vi "Get Cal Proc List.vi"(6 "교정절차 목록 MC List":refnum<vi>, 8 "에러 입력(에러 없음)":errorcluster, 10 "교정정보 in":T1, 11 "참조 번호 입력":T2) -> (0 "에러 출력":errorcluster, 3 "참조 번호 출력":T2, 5 "교정정보 out":T1)   [LabVIEW 2020]
uses:
  <vilib>/addons/database/Connection.llb/Conn ObjectReference.ctl
  Controls/Clst_Cal Info Global.ctl
  Controls/Cmd_Read Query.ctl
  Controls/Clst_Query Info.ctl
  <vilib>/addons/database/NI_Database_API.lvlib
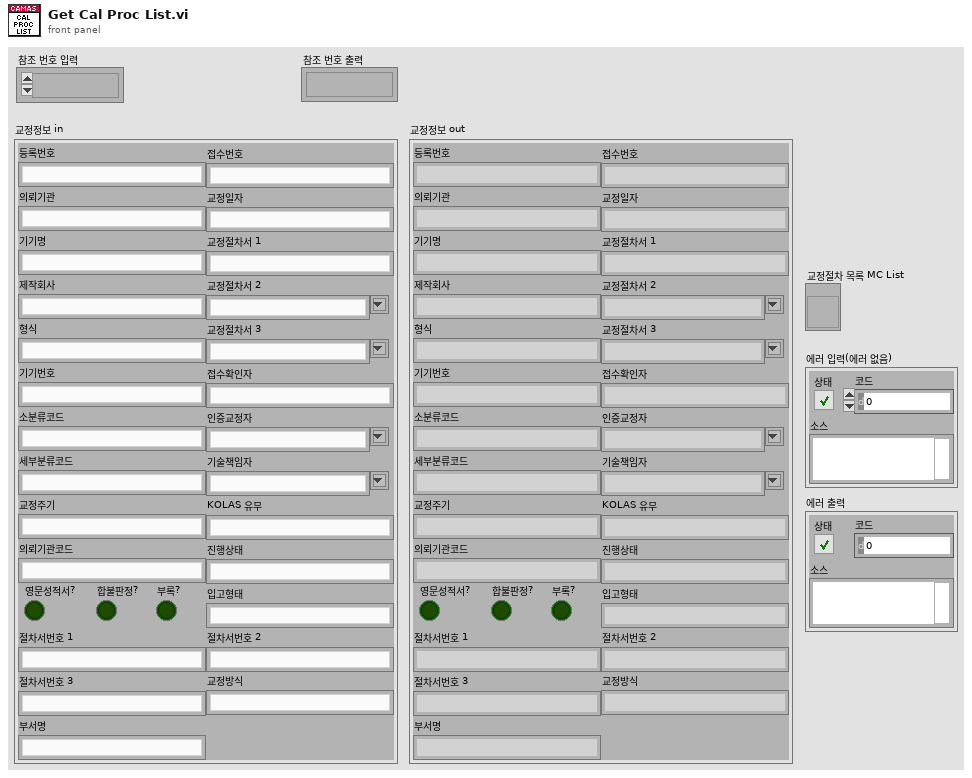
[diagram p1: front panel]
types:
  T1 = typedef "Clst_Cal Info Global.ctl" = cluster{"등록번호":string, "의뢰기관":string, "기기명":string, "제작회사":string, "형식":string, "기기번호":string, "소분류코드":string, "세부분류코드":string, "교정주기":string, "접수번호":string, "교정일자":string, "교정절차서 1":string, "교정절차서 2":string, "교정절차서 3":string, "접수확인자":string, "인증교정자":string, "기술책임자":string, "KOLAS 유무":string, "진행상태":string, "의뢰기관코드":string, "입고형태":string, "영문성적서?":bool, "합불판정?":bool, "부록?":bool, "절차서번호 1":string, "절차서번호 2":string, "절차서번호 3":string, "교정방식":string, "부서명":string}
  T2 = typedef "NI_Database_API.lvlib/Conn ObjectReference.ctl" = refnum<k1>
  T3 = typedef "Clst_Query Info.ctl" = cluster{"사번":string, "등록번호":string, "업체명":string, "세부분류코드":string, "형식":string, "기기번호":string, "FUNC":string, "FUNC_EXT":string, "옵션":string, "추가문자열":string, "일자":string, "배열 1":string[], "배열 2":string[], "항목명":string, "문자열":string, "이름":string}
  T4 = typedef "Cmd_Read Query.ctl" = enum16{"교정자 이름 얻기", "인증교정자 얻기", "기술책임자 얻기", "기책부책 얻기", "등록번호 얻기", "등록정보 얻기", "업체정보 얻기", "교정일자(CAMAS) 얻기", "교정일자(CALSTD) 얻기", "교정환경 얻기", "교정절차서 목록 얻기", "교정절차서명 얻기", "교정절차 목록얻기", "교정절차 얻기", "PROC 교정절차 얻기", "PROC SPEC 얻기", "교정절차(Func별) 얻기", "교정절차(Func_ext별) 얻기", "기관코드 얻기", "교정기능(세부분류) 얻기", "교정기능(모델) 얻기", "교정기능 목록 얻기", "교정기능 명칭 얻기", "교정기능 항목명칭 얻기", "DB (사용기준기) 얻기", "DB (기준기이름) 얻기", "DB (기준기이름목록) 얻기", "DB (기준기목록) 얻기", "DB (기준기값) 얻기", "DB (CMC) 얻기", "DB (FUNC) 얻기", "DB (CALNAME) 얻기", "DB (STDNAME) 얻기", "DB (SPEC) 얻기", "모델(항목전체) 얻기", "모델(최대범위) 얻기", "모델(최소범위) 얻기", "모델(최대최소) 얻기", "모델(범위조건) 얻기", "모델(등록요청) 얻기", "모델(형식별) 얻기", "모델(조건별) 얻기", "모델(모델검색) 얻기", "세부분류 목록 얻기", "기준기등록리스트 얻기", "STD Cal Date Check", "DB등록일자 얻기", "적용항목 얻기", "기타정보 얻기", "기준기요청 얻기", "서버버전 얻기"}
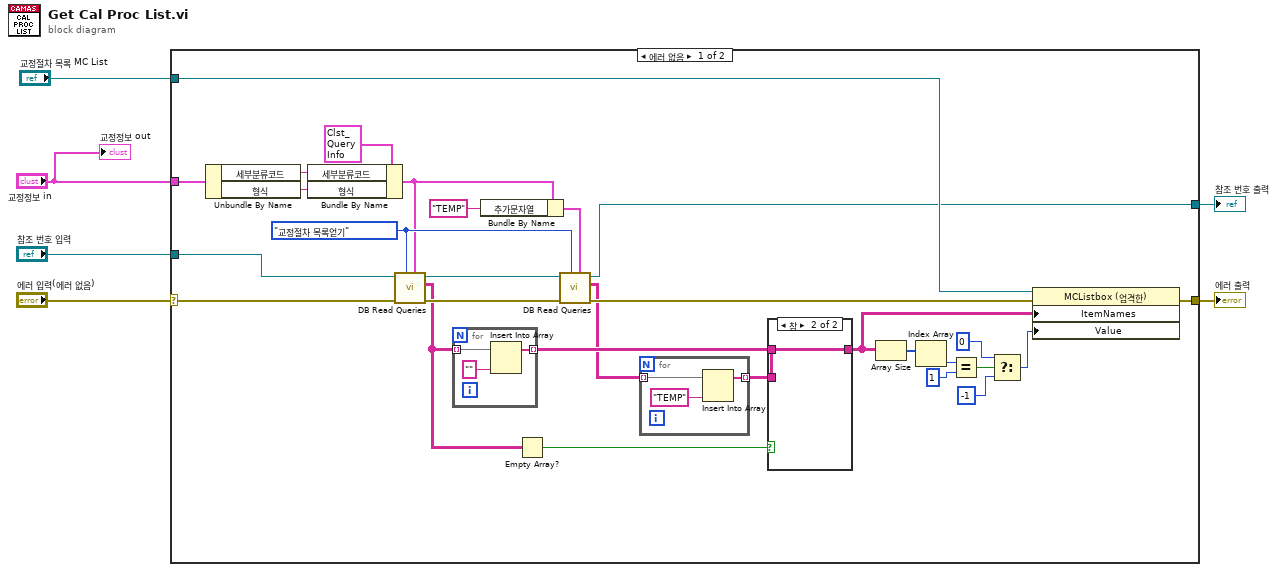
[diagram p0: block diagram]
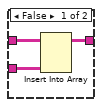
[diagram p2: hidden frame]
diagram:
  n1 = case shown="에러 없음" "에러 입력(에러 없음)" {
    selector: "에러 입력(에러 없음)" -> [w15 w47]
    tunnel: "참조 번호 입력" -> [w35 w46]
    tunnel: [w31 w47] -> w5
    tunnel: "교정절차 목록 MC List" -> [w30 _]
    tunnel: "교정정보 in" -> [w22 _]
    tunnel: [w17 w46] -> w2
    frame No Error {
      w21 = Cmd_Read_Query."교정절차 목록얻기" ("Query Command")
      n2 = Unbundle By Name(w22) -> ("세부분류코드"=w33:string, "형식"=w32:string)
      n3 = Bundle By Name(cluster=T3 {"사번"="", "등록번호"="", "업체명"="", "세부분류코드"="", "형식"="", "기기번호"="", "FUNC"="", "FUNC_EXT"="", "옵션"="", "추가문자열"="", "일자"="", "배열 1"=[], "배열 2"=[], "항목명"="", "문자열"="", "이름"=""} ("Query info"), "세부분류코드"=w33, "형식"=w32) -> (w16:T3)
      n4 = call "DB Read Queries.vi"("Query info"=w16, "Query Command"=w21, "에러 입력(에러 없음)"=w15, "참조 번호 입력"=w35) -> ("에러 출력"=w20:errorcluster, "Data"=w10:string[][], "참조 번호 출력"=w18:T2)  [unwired: 3 in, 2 out]
      n5 = for {
        tunnel: w10 -> [w41] mode=indexing
        tunnel: [w39] -> w9 mode=indexing
        n6 = Insert Into Array(array=w41, new element="") -> (w39:string[])  [unwired: 1 in]
      }
      n7 = Bundle By Name(cluster=w16, "추가문자열"="TEMP") -> (w14:T3)
      n8 = Empty Array?(array=w10) -> (empty?=w11:bool)
      n9 = call "DB Read Queries.vi"("Query info"=w14, "Query Command"=w21, "에러 입력(에러 없음)"=w20, "참조 번호 입력"=w18) -> ("에러 출력"=w19:errorcluster, "Data"=w8:string[][], "참조 번호 출력"=w17:T2)  [unwired: 3 in, 2 out]
      n10 = for {
        tunnel: w8 -> [w38] mode=indexing
        tunnel: [w36] -> w7 mode=indexing
        n11 = Insert Into Array(array=w38, new element="TEMP") -> (w36:string[])  [unwired: 1 in]
      }
      n12 = case shown="참" w11 {
        tunnel: w7 -> [w44 w45]
        tunnel: [w43 w45] -> w12
        tunnel: w9 -> [w42 _]
        frame False {
          n13 = Insert Into Array(array=w42, new element=w44) -> (w43:string[][])  [unwired: 2 in]
        }
        frame True {
        }
      }
      n14 = Array Size(array=w12) -> (size(s)=w29:i32[])
      n15 = Index Array(array=w29) -> (element=w28:i32)  [unwired: 1 in]
      n16 = Equal?(x=w28, y=1) -> (x = y?=w26:bool)
      n17 = Select(t=0, s=w26, f=-1 ("값")) -> (s? t:f=w23:i32)
      n18 = property class="MCListbox (엄격한)"(reference=w30, error in=w19, "ItemNames"=w12, "Value"=w23) -> (error out=w31:errorcluster)  [unwired: 1 out]
    }
    frame Error {
    }
  }
  "참조 번호 출력" <- w2
  "에러 출력" <- w5
  "교정정보 out" <- "교정정보 in"
